vi "Choreo_Util_FieldDimensions.vi"   [LabVIEW 2019, in "ChoreoLib.lvlib"]
uses:
  ChoreoLib.lvlib
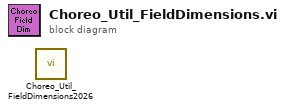
[diagram p0: block diagram]
diagram:
  n1 = call "Choreo_Util_FieldDimensions2026.vi"() -> ()  [unwired: 10 in, 2 out]
